vi "Close.vi"(8 "error in":errorcluster {"code" format="%.0x"}, 11 "UdsHandleIn":T1) -> (0 "error out":errorcluster {"code" format="%.0x"}, 3 "UdsHandleOut":T1)   [LabVIEW 2011, in "Konvolucio MUDS150628.lvlib"]
uses:
  <instrlib>/Konvolucio MUDS150628/Konvolucio MUDS150628.lvlib
  <instrlib>/Konvolucio MUDS150628/Types/UdsHandleType.ctl
  <instrlib>/Konvolucio MCAN120803/Types/MCanHandleType.ctl
  C:/Program Files/National Instruments/LabVIEW 2011/instr.lib/Konvolucio MCAN120803/Private/Konvolucio.MCAN120803.dll
  Konvolucio MCAN120803/Private/Konvolucio.MCAN120803.dll
  <instrlib>/Konvolucio MUDS150628/Private/UdsLogEvent.vi
  <instrlib>/Konvolucio MCAN120803/Konvolucio MCAN120803.lvlib
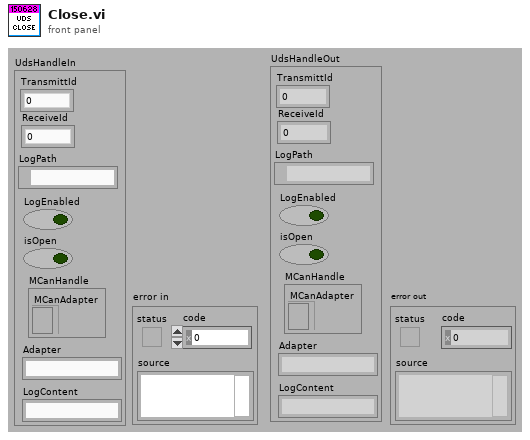
[diagram p1: front panel]
types:
  T1 = typedef "Konvolucio MUDS150628.lvlib/UdsHandleType.ctl" = cluster{"LogPath":path, "LogEnabled":bool, "isOpen":bool, "LogContent":string, "Adapter":string, "MCanHandle":T2, "TransmittId":u32, "ReceiveId":u32}
  T2 = typedef "Konvolucio MCAN120803.lvlib/MCanHandleType.ctl" = cluster{"MCanAdapter":refnum<k24>}
  T3 = enum16{"open", "open or create", "create or replace", "create", "open (read only)"}
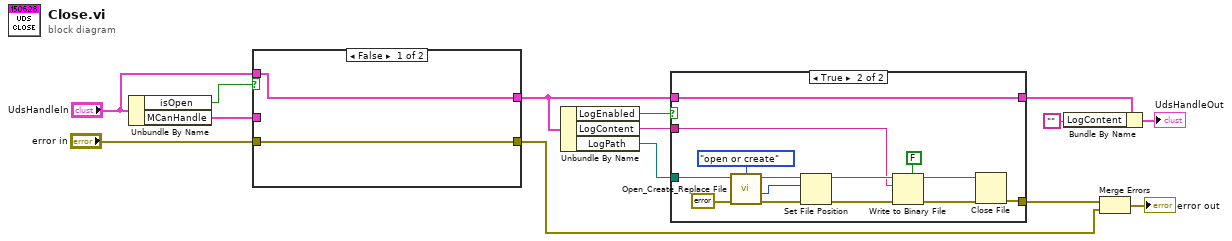
[diagram p0: block diagram]
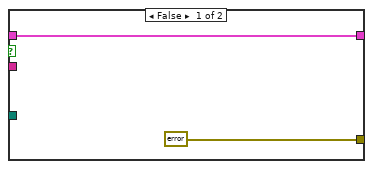
[diagram p2: hidden frame]
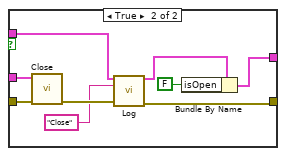
[diagram p3: hidden frame]
diagram:
  n1 = Unbundle By Name("UdsHandleIn") -> ("isOpen"=w5:bool, "MCanHandle"=w14:T2)
  n2 = case shown="False" w5 {
    tunnel: w14 -> [_ w23]
    tunnel: "error in" -> [w16 w24]
    tunnel: [w16 w17] -> w1
    tunnel: [w15 w18] -> w9
    tunnel: "UdsHandleIn" -> [w15 w21]
    frame False {
    }
    frame True {
      n3 = call <instrlib>:"Close.vi"("error in"=w24, "MCanHandleIn"=w23) -> ("error out"=w22:errorcluster)  [unwired: 8 in, 1 out]
      n4 = call-poly <instrlib>:"Log.vi"("UdsHandleIn"=w21, "EventMsg"="Close" ("Request"), "error in"=w22) -> ("UdsHandleOut"=w19:T1, "error out"=w17:errorcluster)  [unwired: 11 in]
      n5 = Bundle By Name(cluster=w19, "isOpen"=FALSE) -> (w18:T1)
    }
  }
  n6 = Unbundle By Name(w9) -> ("LogEnabled"=w3:bool, "LogContent"=w2:string, "LogPath"=w12:path)
  n7 = case shown="True" w3 {
    tunnel: w12 -> [_ w40]
    tunnel: [errorcluster {"status"=FALSE, "code"=0, "source"=""} ("error out") w35] -> w10
    tunnel: w2 -> [_ w29]
    tunnel: [w26 w28] -> w8
    tunnel: w9 -> [w26 w28]
    frame False {
    }
    frame True {
      n8 = call <vilib>:"Open_Create_Replace File.vi"("error in (no error)"=errorcluster {"status"=FALSE, "code"=0, "source"=""}, "function (open:0)"=T3."open or create", "file path"=w40) -> ("error out"=w36:errorcluster, "file size (bytes)"=w37:i32, "refnum"=w38:refnum<file>)  [unwired: 5 in, 1 out]
      n9 = Set File Position(offset (in bytes) (0)=w37, refnum=w38, error in=w36) -> (refnum out=w30:refnum<file>, error out=w33:errorcluster)  [unwired: 1 in]
      n10 = Write to Binary File(file (use dialog)=w30, data=w29, error in=w33, 5:FALSE ("prepend array or string size? (T)")) -> (refnum out=w31:refnum<file>, error out=w32:errorcluster)  [unwired: 2 in, 1 out]
      n11 = Close File(refnum=w31, error in=w32) -> (error out=w35:errorcluster)  [unwired: 1 out]
    }
  }
  n12 = Bundle By Name(cluster=w8, "LogContent"="") -> (→"UdsHandleOut":T1)
  n13 = Merge Errors(w10, w1) -> (→"error out":errorcluster)
